vi "Scale Encoder Counts.vi"(8 "Error In":errorcluster, 9 "Axis Encoder Counts":i32) -> (0 "Error Out":errorcluster, 1 "Axis Encoder Counts out":i32, 2 "Axis Inches":dbl)   [LabVIEW 2013]
doc: "This sub-VI scales encoder counts to inches. Note, 1 encoder count = 1/2000 inches."
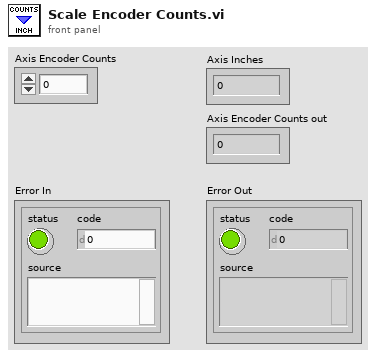
[diagram p1: front panel]
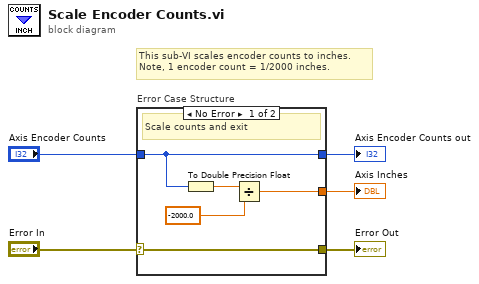
[diagram p0: block diagram]
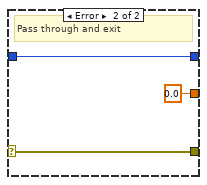
[diagram p2: hidden frame]
diagram:
  # "This sub-VI scales encoder counts to inches.\nNote, 1 encoder count = 1/2000 inches."
  n1 = case "Error Case Structure" shown="No Error" "Error In" {
    selector: "Error In" -> [w7 w11]
    tunnel: "Axis Encoder Counts" -> [w6 w13]
    tunnel: [w8 0.0] -> w4
    tunnel: [w7 w11] -> w2
    tunnel: [w6 w13] -> w1
    frame No Error {
      # "Scale counts and exit"
      n2 = To Double Precision Float(number=w6) -> (double precision float=w9:dbl)
      n3 = Divide(x=w9, y=-2000.0) -> (x/y=w8:dbl)
    }
    frame Error {
      # "Pass through and exit"
    }
  }
  "Axis Encoder Counts out" <- w1
  "Axis Inches" <- w4
  "Error Out" <- w2
